vi "GalvosReset.vi"(8 "error in (no error)":errorcluster, 11 "Microscope in":refnum<class "Microscope.lvclass">) -> (0 "error out":errorcluster, 3 "Microscope out":refnum<class "Microscope.lvclass">)   [LabVIEW 2012, in "Microscope.lvclass"]
uses:
  classes/Microscope.lvclass
  classes/Microscope.lvclass/Microscope.ctl
  <vilib>/DAQmx/write.llb/DAQmx Write (Analog 1D DBL NChan 1Samp).vi
  <vilib>/DAQmx/write.llb/DAQmx Write (Analog 1D Wfm NChan NSamp).vi
  <vilib>/DAQmx/create/channels.llb/DAQmx Create Channel (AO-Voltage-Basic).vi
  <vilib>/DAQmx/configure/timing.llb/DAQmx Timing (Sample Clock).vi
  <vilib>/DAQmx/miscellaneous.llb/DAQmx Fill In Error Info.vi
  <vilib>/DAQmx/configure/trigger.llb/DAQmx Start Trigger (Digital Edge).vi
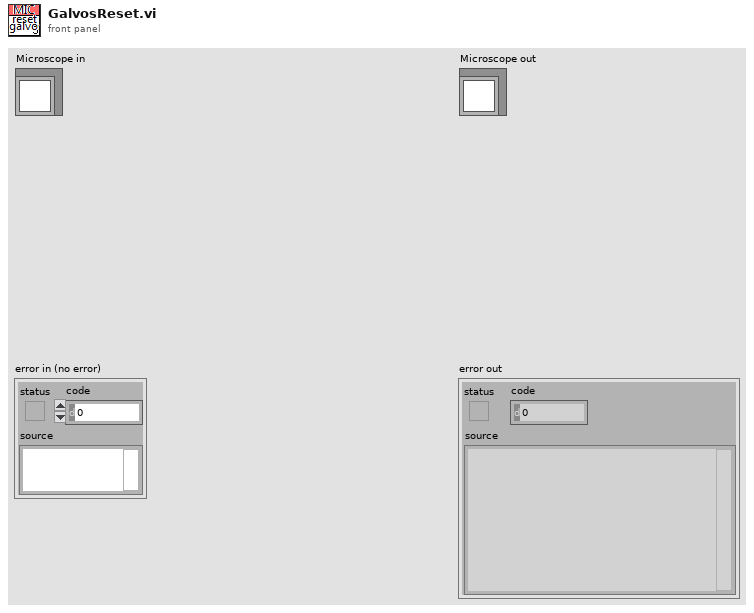
[diagram p1: front panel]
types:
  T1 = typedef "SyncAlgo.ctl" = cluster{"Pixels/sec":dbl, "Pixel Dwell Time (us)":dbl, "Fill Factor":dbl, "Flyback Pixels":dbl, "Lines/sec":dbl, "Galvo Write rate":dbl, "Galvo Timebase divisor":i32, "total pixels per line":dbl, "Samples to Average":dbl, "Trash Samples":dbl, "Actual samples to Read per Line":dbl, "Detector Read rate":dbl, "Detector Timebase divisor":i32}
  T2 = cluster{"x pixels":i32, "x voltage min":dbl, "x voltage max":dbl, "y pixels":i32, "y voltage min":dbl, "y voltage max":dbl, "x pts flyback":i32, "y pts flyback":i32, "Zoom":dbl}
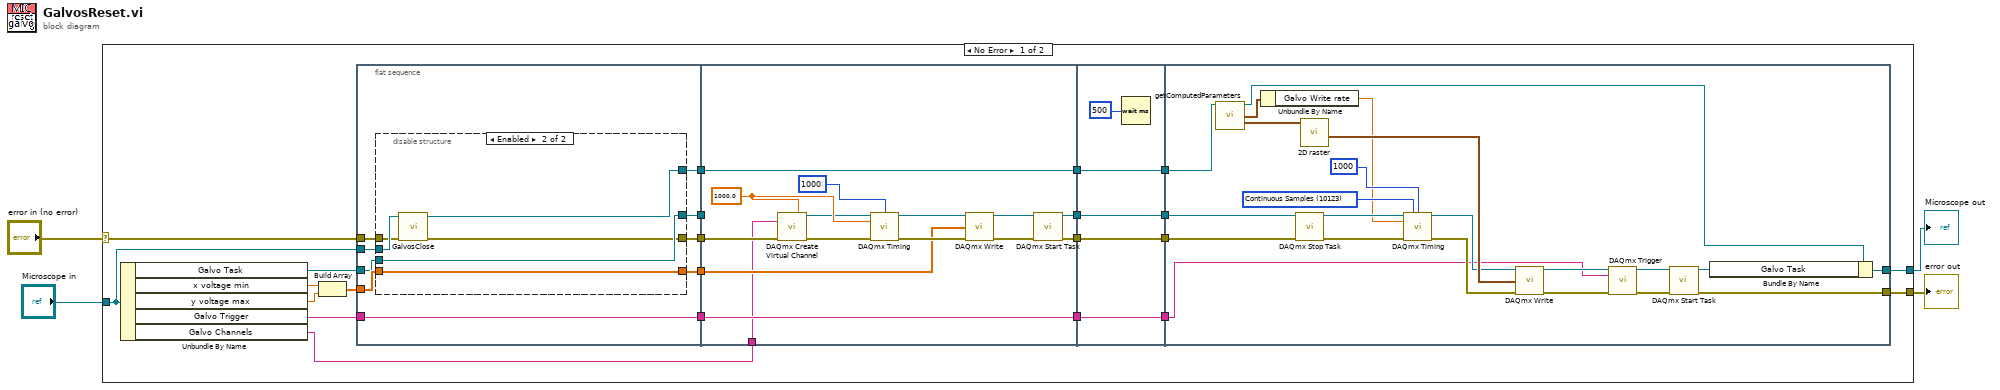
[diagram p0: block diagram]
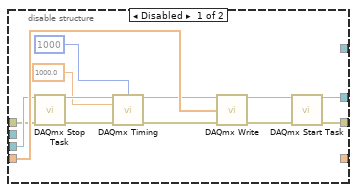
[diagram p2: hidden frame]
diagram:
  n1 = case shown="No Error" "error in (no error)" {
    selector: "error in (no error)" -> [w17 w99]
    tunnel: [w18 w99] -> w3
    tunnel: [w19 w98] -> w2
    tunnel: "Microscope in" -> [w16 w98]
    frame No Error {
      n2 = Unbundle By Name(w16) -> ("Galvo Task"=w27:refnum<k21>, "x voltage min"=w26:dbl, "y voltage max"=w25:dbl, "Galvo Trigger"=w20:tag, "Galvo Channels"=w5:tag)
      n3 = Build Array(w26, w25) -> (w24:dbl[])
      n4 = flat-sequence {
        tunnel: w27 -> [w32]
        tunnel: w24 -> [w36]
        tunnel: [w35] -> w15
        tunnel: [w34] -> w13
        tunnel: [w33] -> w11
        tunnel: w20 -> [w33]
        tunnel: w17 -> [w31]
        tunnel: w16 -> [w30]
        tunnel: [w29] -> w9
        tunnel: [w28] -> w6
        tunnel: w15 -> [_]
        tunnel: [w63] -> w14
        tunnel: w13 -> [w59]
        tunnel: [w61] -> w12
        tunnel: w11 -> [w70]
        tunnel: [w70] -> w10
        tunnel: w9 -> [w64]
        tunnel: [w62] -> w7
        tunnel: w6 -> [w62]
        tunnel: w5 -> [w57]
        tunnel: w14 -> [w74]
        tunnel: [w74] -> w23
        tunnel: [w73] -> w22
        tunnel: w12 -> [w73]
        tunnel: [w72] -> w21
        tunnel: w10 -> [w72]
        tunnel: [w71] -> w8
        tunnel: w7 -> [w71]
        tunnel: w23 -> [w86]
        tunnel: w22 -> [w84]
        tunnel: w21 -> [w87]
        tunnel: [w80] -> w19
        tunnel: [w88] -> w18
        tunnel: w8 -> [w79]
        frame #0 {
          n5 = disable-structure shown="Enabled" {
            disable-tunnel: w36 -> [w49 w54]
            disable-tunnel: [w46 w53] -> w35
            disable-tunnel: [w45 w51] -> w34
            disable-tunnel: w32 -> [w44 w53]
            disable-tunnel: w31 -> [w43 w52]
            disable-tunnel: w30 -> [_ w55]
            disable-tunnel: [_ w54] -> w29
            disable-tunnel: [_ w50] -> w28
            frame Disabled {
              n6 = call <vilib>:"DAQmx Stop Task.vi"("task/channels in"=w44, "error in"=w43) -> ("task out"=w41:refnum<k21>, "error out"=w39:errorcluster)  [unwired: 12 in]
              n7 = call-poly <vilib>:"DAQmx Timing.vi"("task/channels in"=w41, "samples per channel"=1000, "rate"=1000.0, "error in"=w39) -> ("task out"=w40:refnum<k21>, "error out"=w38:errorcluster)  [unwired: 10 in]
              n8 = call-poly <vilib>:"DAQmx Write.vi"("task/channels in"=w40, "data"=w49, "error in"=w38) -> ("task out"=w48:refnum<k21>, "error out"=w47:errorcluster)  [unwired: 10 in, 1 out]
              n9 = call <vilib>:"DAQmx Start Task.vi"("task/channels in"=w48, "error in"=w47) -> ("task out"=w46:refnum<k21>, "error out"=w45:errorcluster)  [unwired: 12 in]
            }
            frame Enabled {
              n10 = call "GalvosClose.vi"("error in (no error)"=w52, "Microscope in"=w55) -> ("error out"=w51:errorcluster, "Microscope out"=w50:refnum<class "Microscope.lvclass">)  [unwired: 8 in]
            }
          }
        }
        frame #1 {
          w60 = 1000.0 ("rate")
          n11 = call-poly <vilib>:"DAQmx Create Virtual Channel.vi"("output terminal configuration"=w60, "physical channels"=w57, "error in"=w59) -> ("task out"=w56:refnum<k21>, "error out"=w58:errorcluster)  [unwired: 11 in]
          n12 = call-poly <vilib>:"DAQmx Timing.vi"("task/channels in"=w56, "samples per channel"=1000, "rate"=w60, "error in"=w58) -> ("task out"=w68:refnum<k21>, "error out"=w69:errorcluster)  [unwired: 10 in]
          n13 = call-poly <vilib>:"DAQmx Write.vi"("task/channels in"=w68, "data"=w64, "error in"=w69) -> ("task out"=w65:refnum<k21>, "error out"=w66:errorcluster)  [unwired: 10 in, 1 out]
          n14 = call <vilib>:"DAQmx Start Task.vi"("task/channels in"=w65, "error in"=w66) -> ("task out"=w63:refnum<k21>, "error out"=w61:errorcluster)  [unwired: 12 in]
        }
        frame #2 {
          n15 = Wait (ms)(milliseconds to wait=u32 500) -> ()  [unwired: 1 out]
        }
        frame #3 {
          w95 = 10123 items=["Finite Samples"=10178, "Continuous Samples"=10123, "Hardware Timed Single Point"=12522] ("sample mode")
          n16 = call "getComputedParameters.vi"("Microscope in"=w79) -> ("Microscope out"=w81:refnum<class "Microscope.lvclass">, "Computed Parameters"=w77:T1, "Scanning Parameters"=w78:T2)  [unwired: 11 in, 1 out]
          n17 = Unbundle By Name(w77) -> ("Galvo Write rate"=w76:dbl)
          n18 = call <vilib>:"DAQmx Stop Task.vi"("task/channels in"=w86, "error in"=w84) -> ("task out"=w85:refnum<k21>, "error out"=w83:errorcluster)  [unwired: 12 in]
          n19 = call "2D raster.vi"("Scanning Parameters"=w78) -> ("X and Y"=w96:waveform(dbl)[])  [unwired: 8 in, 2 out]
          n20 = call-poly <vilib>:"DAQmx Timing.vi"("task/channels in"=w85, "sample mode"=w95, "samples per channel"=1000, "rate"=w76, "error in"=w83) -> ("task out"=w94:refnum<k21>, "error out"=w89:errorcluster)  [unwired: 9 in]
          n21 = call-poly <vilib>:"DAQmx Write.vi"("task/channels in"=w94, "data"=w96, "error in"=w89) -> ("task out"=w93:refnum<k21>, "error out"=w91:errorcluster)  [unwired: 10 in, 1 out]
          n22 = call-poly <vilib>:"DAQmx Trigger.vi"("task/channels in"=w93, "source"=w87, "error in"=w91) -> ("task out"=w92:refnum<k21>, "error out"=w90:errorcluster)  [unwired: 11 in]
          n23 = call <vilib>:"DAQmx Start Task.vi"("task/channels in"=w92, "error in"=w90) -> ("task out"=w82:refnum<k21>, "error out"=w88:errorcluster)  [unwired: 12 in]
          n24 = Bundle By Name(cluster=w81, "Galvo Task"=w82) -> (w80:refnum<class "Microscope.lvclass">)
        }
      }
    }
    frame Error {
    }
  }
  "error out" <- w3
  "Microscope out" <- w2
